vi "serial_write_read.vi"(6 "read byte count":u32=500, 8 "VISA resource name":refnum<visa-resource-name>, 9 "Clear buffer":bool, 11 "write buffer":string="!") -> (0 "VISA resource name out":refnum<visa-resource-name>, 3 "read buffer":string)   [LabVIEW 2021]
panel:
  out "length":i32=1
  out "error out":errorcluster={"status"=TRUE, "code"=-1073807339, "source"="VISA Read in serial_write_read.vi->gantry_rot_stop.vi->MPI2_continious_implementation.vi"}
  out "return count READ":u32
  out "return count WRITE":u32=1
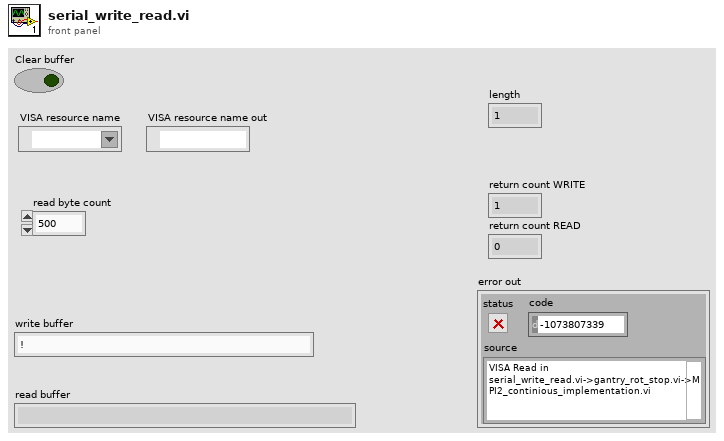
[diagram p1: front panel]
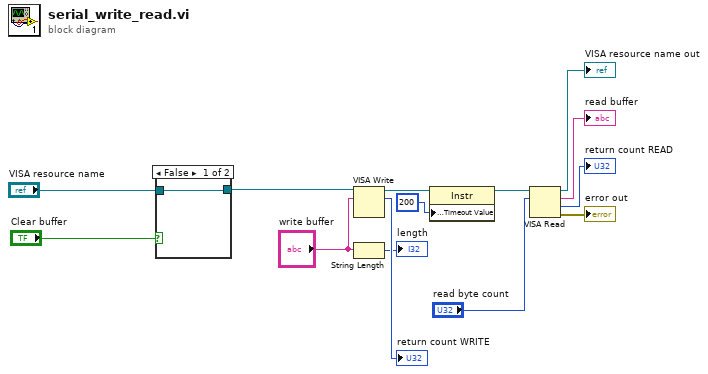
[diagram p0: block diagram]
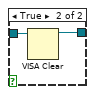
[diagram p2: hidden frame]
diagram:
  n1 = case shown="False" "Clear buffer" {
    tunnel: [w15 w17] -> w3
    tunnel: "VISA resource name" -> [w15 w16]
    frame False {
    }
    frame True {
      n2 = VISA Clear(VISA resource name=w16) -> (VISA resource name out=w17:refnum<visa-resource-name>)  [unwired: 1 in, 1 out]
    }
  }
  n3 = VISA Write(VISA resource name=w3, write buffer="write buffer") -> (VISA resource name out=w8:refnum<visa-resource-name>, return count=→"return count WRITE":u32)  [unwired: 1 in, 1 out]
  n4 = String Length(string="write buffer") -> (length=→"length":i32)
  n5 = property class="Instr"(reference=w8, "General Settings:Timeout Value"=u32 200) -> (reference out=w7:refnum<visa-resource-name>)  [unwired: 1 in, 1 out]
  n6 = VISA Read(VISA resource name=w7, byte count="read byte count") -> (VISA resource name out=→"VISA resource name out":refnum<visa-resource-name>, read buffer=→"read buffer":string, return count=→"return count READ":u32, error out=→"error out":errorcluster)  [unwired: 1 in]
